vi "Untitled 1 (SubVI).vi"(0 "NeedleValve in":refnum<class "NeedleValve.lvclass">, 11 "error in (no error)":errorcluster) -> (4 "NeedleValve out":refnum<class "NeedleValve.lvclass">, 15 "error out":errorcluster)   [LabVIEW 2019]
uses:
  NeedleValve.lvclass
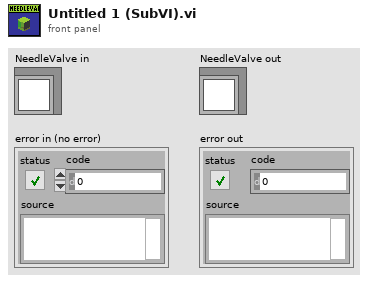
[diagram p1: front panel]
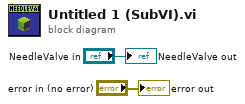
[diagram p0: block diagram]
diagram:
  "NeedleValve out" <- "NeedleValve in"
  "error out" <- "error in (no error)"
